vi "Convert_v00.vi"(8 "Extras PII":T1, 11 "PII Control":T2={"Offset Error"=-0.08983050847457627, "Gain Error"=1, "Offset DC"=-0.003954802259887008, "Gain DC"=1, "P Gain"=20, "P Bit Shift"=-12, "I Bit Shift"=-12, "I2 Bit Shift"=-27, "I Gain"=20, "I2 Gain"=0, "Lock Threshold"=45, "Lock"=FALSE, "Hold"=FALSE, "Scan Frequency"=10, "Scan Bit Shift"=-4, "DC negative"=FALSE, "Gains -ve "=FALSE} {"Scan Frequency" scale=1.0..30.0; "I2 Gain" scale=0.0..10.0; "I Gain" scale=0.0..50.0; "P Gain" scale=0.0..50.0; "Offset DC" scale=-0.1..0.1 scale format="%#_5f"; "Offset Error" scale=-0.1..0.1 scale format="%#_5f"}) -> (3 "PII+Error":T12)   [LabVIEW 2011]
uses:
  Strict Type Defs/PII individual.ctl
  Strict Type Defs/Errors Converted.ctl
  Strict Type Defs/Controls Converted.ctl
  Strict Type Defs/Control GUI v01.ctl
  Strict Type Defs/Slider and display.ctl
  Strict Type Defs/I16 white control.ctl
  Strict Type Defs/PII Gains.ctl
  Strict Type Defs/I2 gain slider.ctl
  Strict Type Defs/Thresh slider.ctl
  Strict Type Defs/Lock or Hold.ctl
  Strict Type Defs/Scan Freq Slider.ctl
  Strict Type Defs/DC polarity.ctl
  Strict Type Defs/Gains negative horizontal.ctl
  Strict Type Defs/Extras PII.ctl
panel:
  in  "PII+Error":T12
  in  "Error individual":T13
  in  "PII In typdef":T14
  # "PII Gains"
  # "Lock"
  # "Error Signal"
  # "Monitor"
  # "Scan"
  # "DC positive"
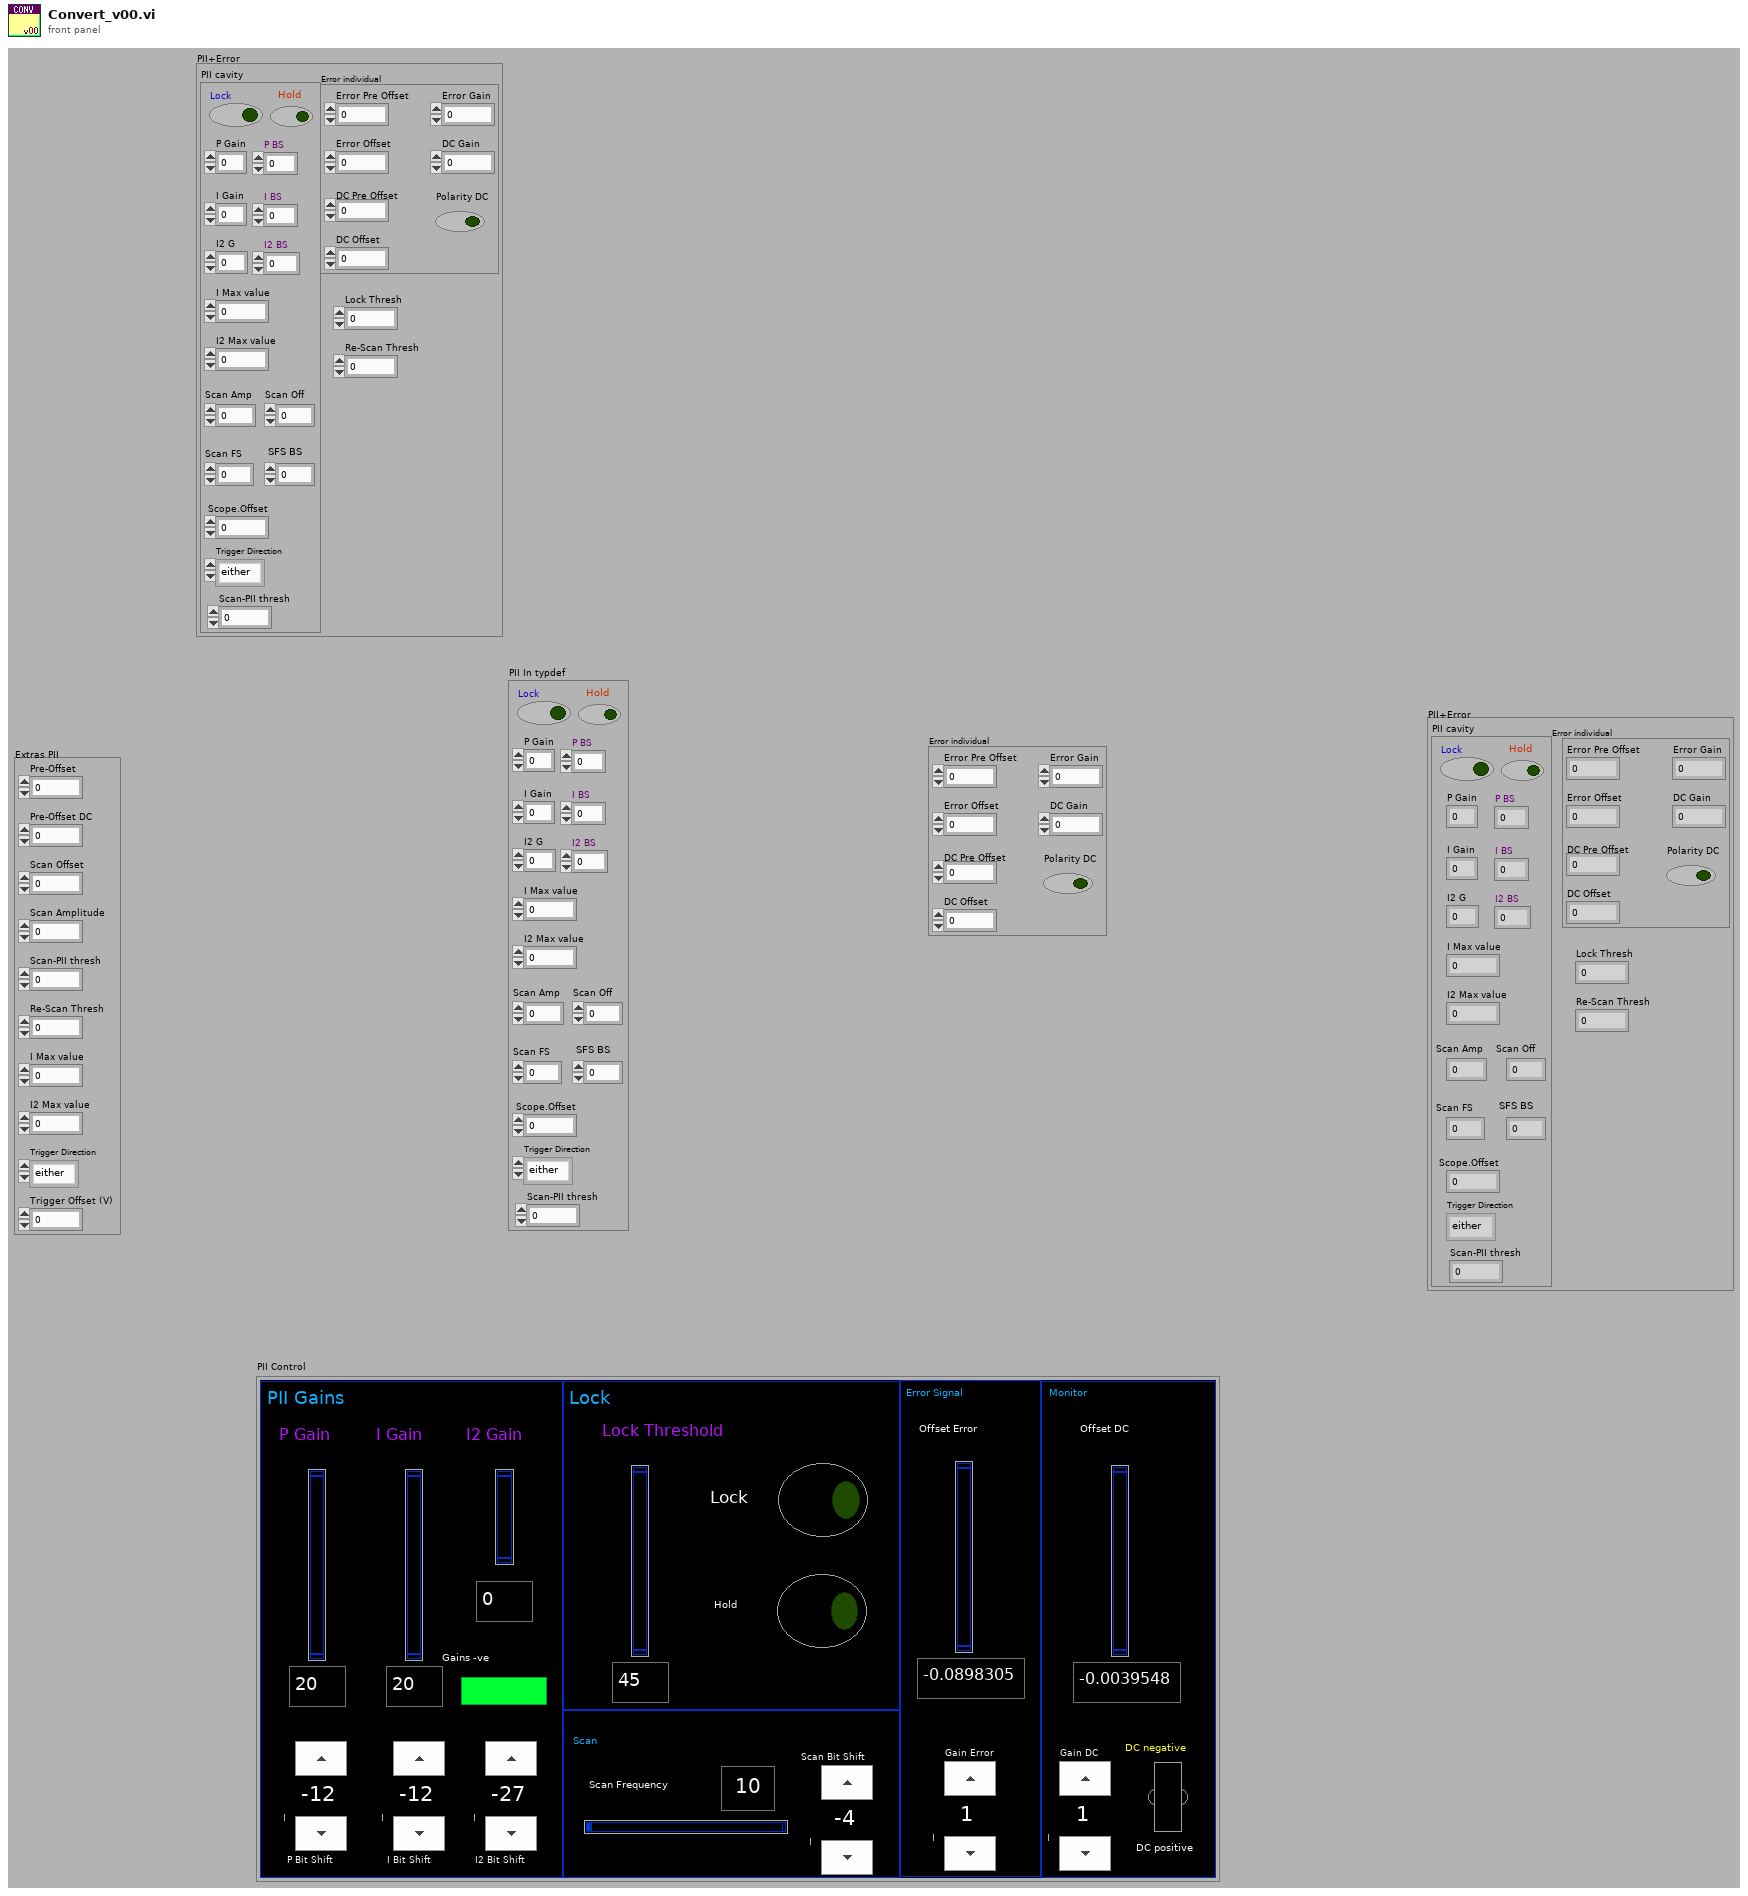
[diagram p1: front panel]
types:
  T1 = typedef "Extras PII.ctl" = cluster{"Pre-Offset":dbl, "Pre-Offset DC":dbl, "Scan Offset":dbl, "Scan Amplitude":dbl, "Scan-PII thresh":i16, "Re-Scan Thresh":i16, "I Max value":i32, "I2 Max value":i32, "Trigger Direction":enum8{"either", "minus-plus", "plus-minus"}, "Trigger Offset (V)":dbl}
  T2 = typedef "Control GUI v01.ctl" = cluster{"Offset Error":T3, "Gain Error":T4, "Offset DC":T3, "Gain DC":T4, "P Gain":T5, "P Bit Shift":T4, "I Bit Shift":T4, "I2 Bit Shift":T4, "I Gain":T5, "I2 Gain":T6, "Lock Threshold":T7, "Lock":T8, "Hold":T8, "Scan Frequency":T9, "Scan Bit Shift":T4, "DC negative":T10, "Gains -ve ":T11}
  T3 = typedef "Slider and display.ctl" = dbl
  T4 = typedef "I16 white control.ctl" = i16
  T5 = typedef "PII Gains.ctl" = i32
  T6 = typedef "I2 gain slider.ctl" = i32
  T7 = typedef "Thresh slider.ctl" = i16
  T8 = typedef "Lock or Hold.ctl" = bool
  T9 = typedef "Scan Freq Slider.ctl" = u16
  T10 = typedef "DC polarity.ctl" = bool
  T11 = typedef "Gains negative horizontal.ctl" = bool
  T12 = typedef "Controls Converted.ctl" = cluster{"Error individual":T13, "PII cavity":T14, "Lock Thresh":i16, "Re-Scan Thresh":i16}
  T13 = typedef "Errors Converted.ctl" = cluster{"Error Pre Offset":i16, "Error Offset":i16, "DC Pre Offset":i16, "DC Offset":i16, "Polarity DC":bool, "Error Gain":i16, "DC Gain":i16}
  T14 = typedef "PII individual.ctl" = cluster{"Lock":bool, "Hold":bool, "P Gain":i32, "P BS":i16, "I Gain":i32, "I BS":i16, "I2 G":i32, "I2 BS":i16, "Scan Amp":i16, "Scan Off":i16, "Scan FS":u16, "SFS BS":i16, "I Max value":i32, "I2 Max value":i32, "Scope.Offset":i16, "Trigger Direction":enum8{"either", "minus-plus", "plus-minus"}, "Scan-PII thresh":i16}
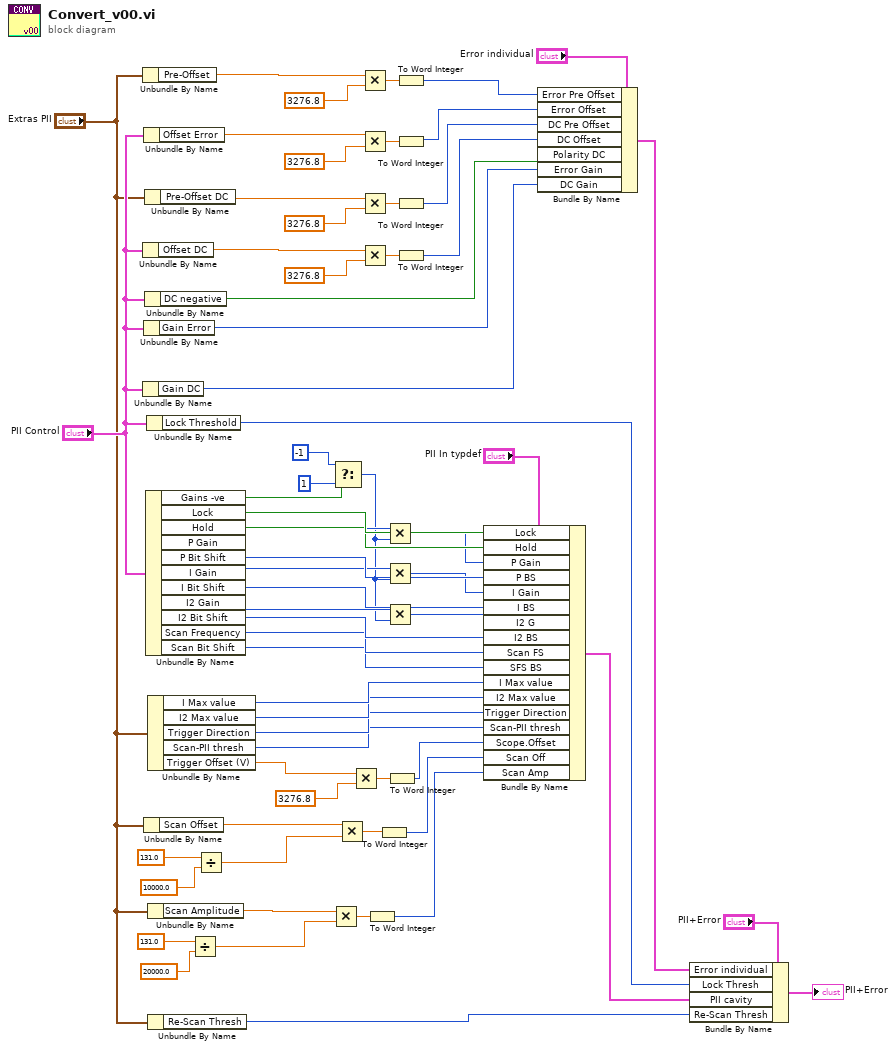
[diagram p0: block diagram]
diagram:
  n1 = Unbundle By Name("Extras PII") -> ("Pre-Offset"=w15:dbl)
  n2 = Unbundle By Name("PII Control") -> ("Offset DC"=w56:T3)
  n3 = Unbundle By Name("PII Control") -> ("Gain DC"=w18:T4)
  n4 = Unbundle By Name("PII Control") -> ("Offset Error"=w62:T3)
  n5 = Unbundle By Name("PII Control") -> ("Gain Error"=w19:T4)
  n6 = Unbundle By Name("Extras PII") -> ("Scan Offset"=w14:dbl)
  n7 = Unbundle By Name("Extras PII") -> ("Pre-Offset DC"=w57:dbl)
  n8 = Unbundle By Name("PII Control") -> ("DC negative"=w23:T10)
  n9 = Unbundle By Name("PII Control") -> ("Gains -ve"=w40:T11, "Lock"=w45:T8, "Hold"=w44:T8, "P Gain"=w39:T5, "P Bit Shift"=w43:T4, "I Gain"=w35:T5, "I Bit Shift"=w42:T4, "I2 Gain"=w33:T6, "I2 Bit Shift"=w41:T4, "Scan Frequency"=w30:T9, "Scan Bit Shift"=w29:T4)
  n10 = Unbundle By Name("PII Control") -> ("Lock Threshold"=w12:T7)
  n11 = Unbundle By Name("Extras PII") -> ("I Max value"=w9:i32, "I2 Max value"=w8:i32, "Trigger Direction"=w7:enum8{"either", "minus-plus", "plus-minus"}, "Scan-PII thresh"=w6:i16, "Trigger Offset (V)"=w2:dbl)
  n12 = Unbundle By Name("Extras PII") -> ("Scan Amplitude"=w55:dbl)
  n13 = Unbundle By Name("Extras PII") -> ("Re-Scan Thresh"=w13:i16)
  n14 = Divide(x=131.0, y=20000.0) -> (x/y=w50:dbl)
  n15 = Divide(x=131.0, y=10000.0) -> (x/y=w47:dbl)
  n16 = Multiply(x=w55, y=w50) -> (x*y=w53:dbl)
  n17 = Select(t=T5 -1 ("y"), s=w40, f=T5 1) -> (s? t:f=w31:T5)
  n18 = Multiply(x=w14, y=w47) -> (x*y=w54:dbl)
  n19 = Multiply(x=w2, y=3276.8) -> (x*y=w4:dbl)
  n20 = Multiply(x=w15, y=3276.8) -> (x*y=w65:dbl)
  n21 = Multiply(x=w62, y=3276.8) -> (x*y=w64:T3)
  n22 = Multiply(x=w57, y=3276.8) -> (x*y=w59:dbl)
  n23 = Multiply(x=w56, y=3276.8) -> (x*y=w60:T3)
  n24 = To Word Integer(number=w53) -> (16bit integer=w11:i16)
  n25 = To Word Integer(number=w54) -> (16bit integer=w5:i16)
  n26 = Multiply(x=w39, y=w31) -> (x*y=w36:T5)
  n27 = Multiply(x=w35, y=w31) -> (x*y=w34:T5)
  n28 = Multiply(x=w33, y=w31) -> (x*y=w32:T6)
  n29 = To Word Integer(number=w4) -> (16bit integer=w1:i16)
  n30 = To Word Integer(number=w65) -> (16bit integer=w27:i16)
  n31 = To Word Integer(number=w64) -> (16bit integer=w26:i16)
  n32 = To Word Integer(number=w59) -> (16bit integer=w25:i16)
  n33 = To Word Integer(number=w60) -> (16bit integer=w24:i16)
  n34 = Bundle By Name(cluster="PII In typdef", "Lock"=w45, "Hold"=w44, "P Gain"=w36, "P BS"=w43, "I Gain"=w34, "I BS"=w42, "I2 G"=w32, "I2 BS"=w41, "Scan FS"=w30, "SFS BS"=w29, "I Max value"=w9, "I2 Max value"=w8, "Trigger Direction"=w7, "Scan-PII thresh"=w6, "Scope.Offset"=w1, "Scan Off"=w5, "Scan Amp"=w11) -> (w20:T14)
  n35 = Bundle By Name(cluster="Error individual", "Error Pre Offset"=w27, "Error Offset"=w26, "DC Pre Offset"=w25, "DC Offset"=w24, "Polarity DC"=w23, "Error Gain"=w19, "DC Gain"=w18) -> (w21:T13)
  n36 = Bundle By Name(cluster="PII+Error", "Error individual"=w21, "Lock Thresh"=w12, "PII cavity"=w20, "Re-Scan Thresh"=w13) -> (→"PII+Error":T12)
